vi "send_burleighJumpTrain-v02.vi"(0 "daq_ao":tag="Dev1/ao1", 1 "daq_ai":tag="Dev1/ai0:1", 2 "Jump Polarity":bool, 5 "JumpTrainValuesCluster":T2, 7 "Sample Freq (Hz)":dbl min=0.0 max=40000.0, 12 "Jump Filter Freq (Hz)":dbl=20.0 min=0.0 max=40000.0, 13 "Number of Replicates":i16=1 min=1 max=10, 14 "error in":errorcluster) -> (4 "output cluster":T1, 6 "output waveform":waveform(dbl)(graph), 8 "protocol response":waveform(dbl)[](graph) caption="jumptestMonitor", 10 "error out":errorcluster)   [LabVIEW 2019]
uses:
  <vilib>/Analysis/3filter.llb/Filter Passband Type.ctl
  <vilib>/Analysis/3filter.llb/Bessel Filter (DBL).vi
  <vilib>/measure/NI_MABase.lvlib
  <vilib>/Analysis/NI_AALBase.lvlib
panel:
  # "Low"
  # "High"
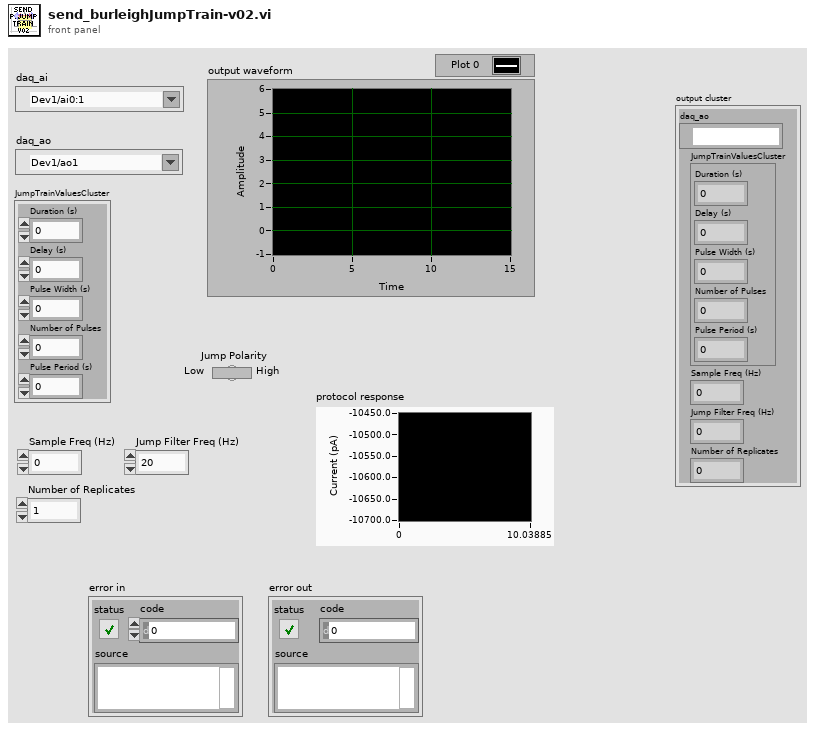
[diagram p1: front panel]
types:
  T1 = cluster{"daq_ao":tag, "JumpTrainValuesCluster":cluster{"Duration (s)":dbl, "Delay (s)":dbl, "Pulse Width (s)":dbl, "Number of Pulses":dbl, "Pulse Period (s)":dbl}, "Sample Freq (Hz)":dbl, "Jump Filter Freq (Hz)":dbl, "Number of Replicates":i16}
  T2 = cluster{"Duration (s)":dbl, "Delay (s)":dbl, "Pulse Width (s)":dbl, "Number of Pulses":dbl, "Pulse Period (s)":dbl}
  T3 = typedef "NI_AALBase.lvlib/Filter Passband Type.ctl" = enum32{"Lowpass", "Highpass", "Bandpass", "Bandstop"}
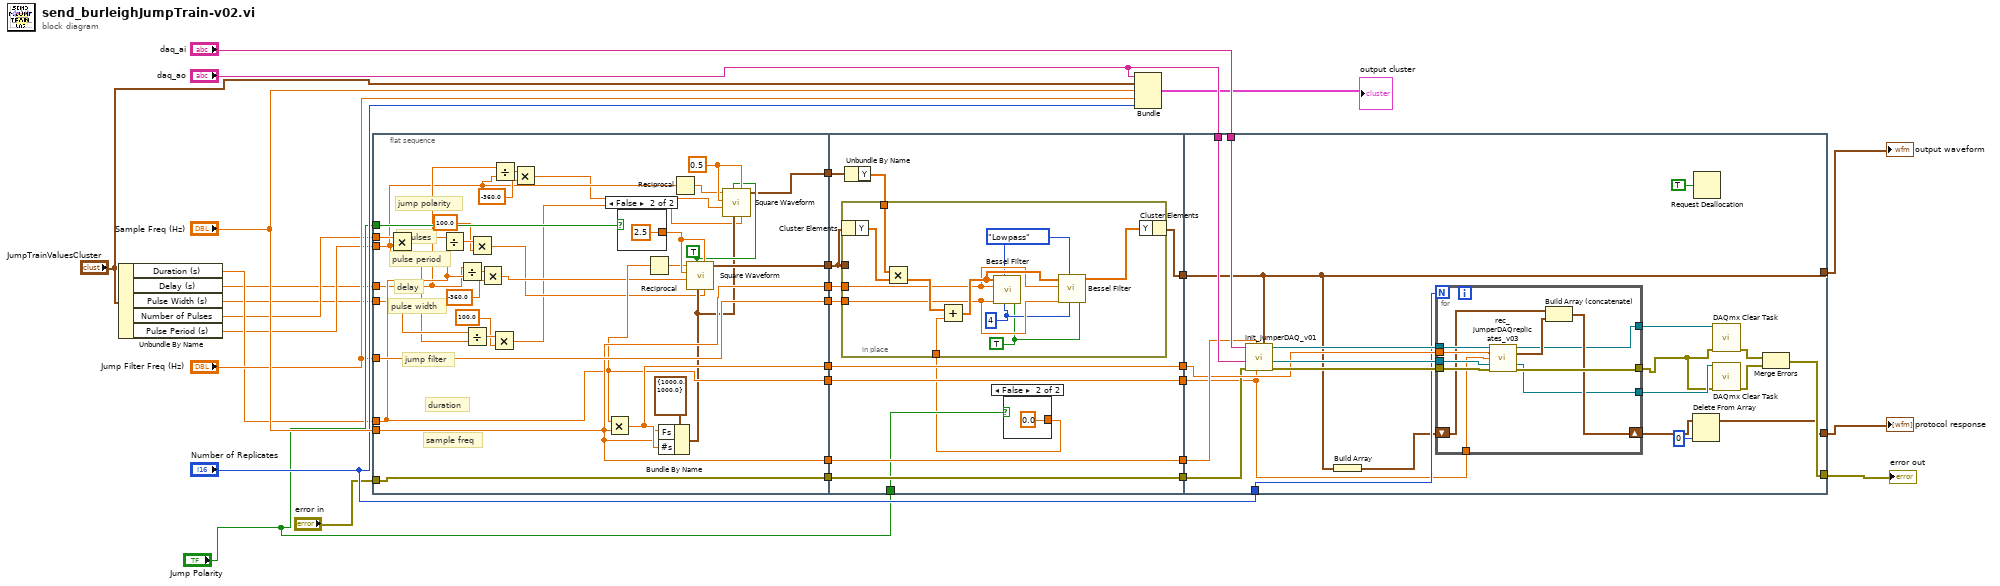
[diagram p0: block diagram]
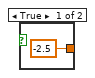
[diagram p2: hidden frame]
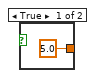
[diagram p3: hidden frame]
diagram:
  n1 = Unbundle By Name("JumpTrainValuesCluster") -> ("Duration (s)"=w7:dbl, "Delay (s)"=w4:dbl, "Pulse Width (s)"=w3:dbl, "Number of Pulses"=w6:dbl, "Pulse Period (s)"=w5:dbl)
  n2 = flat-sequence {
    tunnel: w7 -> [w50]
    tunnel: "Jump Filter Freq (Hz)" -> [w60]
    tunnel: "Sample Freq (Hz)" -> [w59]
    tunnel: [w61] -> w25
    tunnel: [w59] -> w22
    tunnel: [w60] -> w20
    tunnel: [w59] -> w19
    tunnel: [w58] -> w18
    tunnel: "error in" -> [w57]
    tunnel: [w57] -> w14
    tunnel: "Jump Polarity" -> [w56]
    tunnel: [w50] -> w10
    tunnel: w6 -> [w48]
    tunnel: w5 -> [w32]
    tunnel: w4 -> [w33]
    tunnel: w3 -> [w41]
    tunnel: [w40] -> w2
    tunnel: w25 -> [w76]
    tunnel: [w76] -> w24
    tunnel: [w65] -> w23
    tunnel: w22 -> [w75]
    tunnel: [w75] -> w21
    tunnel: w20 -> [w67]
    tunnel: w19 -> [w68]
    tunnel: w18 -> [w66]
    tunnel: [w74] -> w15
    tunnel: w14 -> [w74]
    tunnel: "Jump Polarity" -> [w73]
    tunnel: w10 -> [w72]
    tunnel: [w72] -> w9
    tunnel: w2 -> [w70]
    tunnel: [w91] -> w30
    tunnel: w24 -> [w105]
    tunnel: w23 -> [w91]
    tunnel: "daq_ai" -> [w108]
    tunnel: "daq_ao" -> [w107]
    tunnel: w21 -> [w106]
    tunnel: [w94] -> w27
    tunnel: "Number of Replicates" -> [w104]
    tunnel: [w98] -> w13
    tunnel: w15 -> [w103]
    tunnel: w9 -> [w92]
    frame #0 {
      w46 = 0.5 ("Amplitude")
      w45 = TRUE ("reset signal")
      # "sample freq"
      # "duration"
      # "jump filter"
      # "pulse width"
      # "delay"
      # "pulse period"
      # "#pulses"
      # "jump polarity"
      n3 = Multiply(x=w48, y=w32) -> (x*y=w49:dbl)
      n4 = Divide(x=w49, y=w50) -> (x/y=w54:dbl)
      n5 = Divide(x=w33, y=w50) -> (x/y=w51:dbl)
      n6 = Divide(x=w41, y=w32) -> (x/y=w43:dbl)
      n7 = Multiply(x=w54, y=100.0) -> (x*y=w37:dbl)
      n8 = Multiply(x=w51, y=-360.0) -> (x*y=w44:dbl)
      n9 = Multiply(x=w43, y=100.0) -> (x*y=w36:dbl)
      n10 = Divide(x=w33, y=w32) -> (x/y=w35:dbl)
      n11 = Multiply(x=w35, y=-360.0) -> (x*y=w31:dbl)
      n12 = Multiply(x=w50, y=w59) -> (x*y=w61:dbl)
      n13 = case shown="False" w56 {
        tunnel: [-2.5 ("Amplitude") 2.5 ("Amplitude")] -> w55
        frame True {
        }
        frame False {
        }
      }
      n14 = Reciprocal(x=w50) -> (1/x=w47:dbl)
      n15 = Bundle By Name(cluster=cluster{"Fs":dbl, "#s":dbl} {"Fs"=1000.0, "#s"=1000.0} ("sampling info"), "Fs"=w59, "#s"=w61) -> (w39:cluster{"Fs":dbl, "#s":dbl})
      n16 = Reciprocal(x=w32) -> (1/x=w38:dbl)
      n17 = call <vilib>:"Square Waveform.vi"("duty cycle (%)"=w37, "offset"=w55, "sampling info"=w39, "reset signal"=w45, "phase"=w44, "amplitude"=w55, "frequency"=w47) -> ("signal out"=w58:waveform(dbl))  [unwired: 3 in, 1 out]
      n18 = call <vilib>:"Square Waveform.vi"("duty cycle (%)"=w36, "offset"=w46, "sampling info"=w39, "reset signal"=w45, "phase"=w31, "amplitude"=w46, "frequency"=w38) -> ("signal out"=w40:waveform(dbl))  [unwired: 3 in, 1 out]
    }
    frame #1 {
      n19 = Unbundle By Name(w70) -> ("Y"=w69:dbl[])
      n20 = case shown="False" w73 {
        tunnel: [5.0 ("Amplitude") 0.0 ("Amplitude")] -> w71
        frame True {
        }
        frame False {
        }
      }
      n21 = in-place {
        in-place-border: w66 -> [_]
        in-place-border: w71 -> [w87]
        in-place-border: w69 -> [w86]
        in-place-border: w68 -> [w83]
        in-place-border: w67 -> [w82]
        w80 = TRUE ("init/cont (init:F)")
        w81 = 4 ("order")
        w79 = Filter_Passband_Type."Lowpass" ("filter type")
        n22 = in-place-cluster #1(w66) -> ("Y"=w77:dbl[])
        n23 = Multiply(x=w86, y=w77) -> (x*y=w85:dbl[])
        n24 = Add(x=w85, y=w87) -> (x+y=w84:dbl[])
        n25 = call-poly <vilib>:"Bessel Filter.vi"("init/cont (init:F)"=w80, "order"=w81, "filter type"=w79, "low cutoff freq: fl"=w82, "sampling freq: fs"=w83, "X"=w84) -> ()  [unwired: 2 in, 2 out]
        n26 = call-poly <vilib>:"Bessel Filter.vi"("init/cont (init:F)"=w80, "order"=w81, "filter type"=w79, "low cutoff freq: fl"=w82, "sampling freq: fs"=w83, "X"=w84) -> ("Filtered X"=w78:dbl[])  [unwired: 2 in, 1 out]
        n27 = in-place-cluster #1("Y"=w78) -> (w65:waveform(dbl))
      }
    }
    frame #2 {
      n28 = call "init_jumperDAQ_v01.vi"("protocol waveform"=w91, "Duration (s)"=w92, "Sample Freq (Hz)"=w106, "AO error in"=w103, "AO physical channels"=w107, "AI Physical Channel"=w108) -> ("AO error out"=w111:errorcluster, "AO task out"=w110:refnum<k21>, "AI task out"=w109:refnum<k21>)  [unwired: 1 in, 2 out]
      n29 = Build Array(w91) -> (w96:waveform(dbl)[])
      n30 = for {
        N: w104 -> [_]
        tunnel: w111 -> [w122]
        tunnel: w110 -> [w121]
        tunnel: w109 -> [w120]
        tunnel: w105 -> [w118]
        shift-right: [w116] -> w95
        shift-left: w96 -> [w115]
        tunnel: [w119] -> w100
        tunnel: [w114] -> w102
        tunnel: [w113] -> w101
        tunnel: w92 -> [w112]
        n31 = call "rec_jumperDAQreplicates_v03.vi"("AI task in"=w120, "number of samples"=w118, "Duration (s)"=w112, "AO task in"=w121, "error in"=w122) -> ("AI task out"=w113:refnum<k21>, "data out (pA or mV)"=w117:waveform(dbl), "AO task out"=w114:refnum<k21>, "error out"=w119:errorcluster)  [unwired: 7 in]
        n32 = Build Array (concatenate)(w115, w117) -> (w116:waveform(dbl)[])
      }
      n33 = Delete From Array(array=w95, index=0) -> (array with subset deleted=w94:waveform(dbl)[])  [unwired: 1 in, 1 out]
      n34 = Request Deallocation(TRUE ("flag")) -> ()
      n35 = call <vilib>:"DAQmx Clear Task.vi"("task in"=w101, "error in"=w100) -> ("error out"=w97:errorcluster)  [unwired: 13 in]
      n36 = call <vilib>:"DAQmx Clear Task.vi"("task in"=w102, "error in"=w100) -> ("error out"=w99:errorcluster)  [unwired: 13 in]
      n37 = Merge Errors(w97, w99) -> (w98:errorcluster)
    }
  }
  n38 = Bundle("daq_ao"="daq_ao", "JumpTrainValuesCluster"="JumpTrainValuesCluster", "Sample Freq (Hz)"="Sample Freq (Hz)", "Jump Filter Freq (Hz)"="Jump Filter Freq (Hz)", "Number of Replicates"="Number of Replicates") -> (→"output cluster":T1)  [unwired: 1 in]
  "protocol response" <- w27
  "output waveform" <- w30
  "error out" <- w13
